vi "Get ESP Template Path.vi"(0 "LabVIEW Web Service Request":refnum<class "Web Request.lvclass">, 5 "Relative Template Path":path, 11 "error in (no error)":errorcluster) -> (4 "LabVIEW Web Service Request out":refnum<class "Web Request.lvclass">, 6 "Template Name":string, 15 "error out":errorcluster)   [LabVIEW 2018]
doc: "This VI determines the path to an ESP template stored in the web service's private folder."
uses:
  <vilib>/wsapi/Web Request.lvclass
  C:/Program Files/National Instruments/LabVIEW 2018/vi.lib/wsapi/Web Service.lvclass
  <vilib>/wsapi/Web Service.lvclass
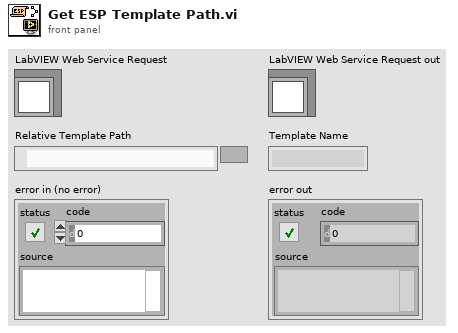
[diagram p1: front panel]
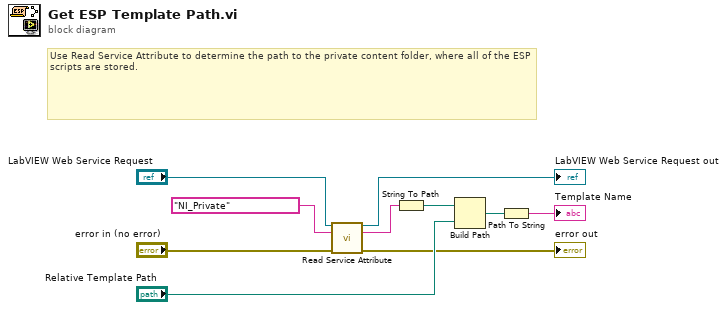
[diagram p0: block diagram]
diagram:
  # "Use Read Service Attribute to determine the path to the private content folder, where all of the ESP scripts are stored."
  n1 = call <vilib>:"Read Service Attribute.vi"("LabVIEW Web Service"="LabVIEW Web Service Request", "attribute name"="NI_Private", "error in (no error)"="error in (no error)") -> ("LabVIEW Web Service out"=→"LabVIEW Web Service Request out":refnum<class "Web Request.lvclass">, "value"=w7:string, "error out"=→"error out":errorcluster)  [unwired: 10 in]
  n2 = String To Path(string=w7) -> (path=w6:path)
  n3 = Build Path(base path=w6, name or relative path="Relative Template Path") -> (appended path=w2:path)
  n4 = Path To String(path=w2) -> (string=→"Template Name":string)
